vi "Read Measurement (Occupied Bandwidth).vi"(0 "VISA resource name":refnum<visa-resource-name>, 5 "Maximum Time (120000 ms)":i32=120000, 11 "error in (no error)":errorcluster) -> (4 "VISA resource name out":refnum<visa-resource-name>, 6 "Occupied Bandwidth(Hz)":dbl, 10 "Centroid Bandwidth(Hz)":dbl, 15 "error out":errorcluster)   [LabVIEW 2022 SP3, in "Agilent N934X Series.lvlib"]
doc: "Reads the measurement result from the spectrum analyzer (Occupied Bandwidth Measurement)."
uses:
  <instrlib>/Agilent N934X Series/Agilent N934X Series.lvlib
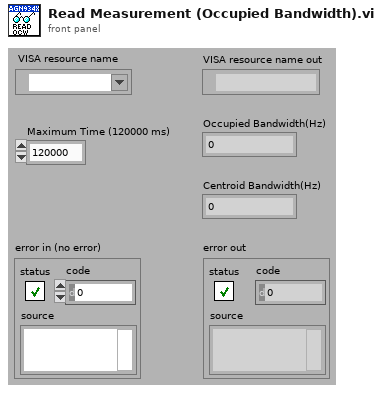
[diagram p1: front panel]
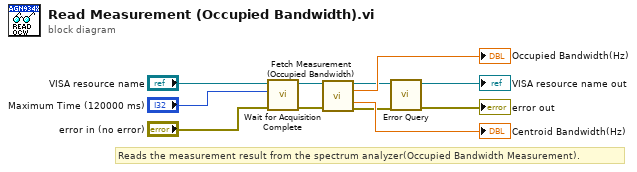
[diagram p0: block diagram]
diagram:
  # "Reads the measurement result from the spectrum analyzer(Occupied Bandwidth Measurement)."
  n1 = call <instrlib>:"Wait for Acquisition Complete.vi"("error in (no error)"="error in (no error)", "Maximum Time (10000 ms)"="Maximum Time (120000 ms)", "VISA resource name"="VISA resource name") -> ("error out"=w6:errorcluster, "VISA resource name out"=w8:refnum<visa-resource-name>)  [unwired: 7 in]
  n2 = call <instrlib>:"Fetch Measurement (Occupied Bandwidth).vi"("VISA resource name"=w8, "error in (no error)"=w6) -> ("VISA resource name out"=w4:refnum<visa-resource-name>, "Occupied Bandwidth(Hz)"=→"Occupied Bandwidth(Hz)":dbl, "Centroid Bandwidth(Hz)"=→"Centroid Bandwidth(Hz)":dbl, "error out"=w3:errorcluster)  [unwired: 10 in]
  n3 = call <instrlib>:"Error Query.vi"("error in (no error)"=w3, "VISA resource name"=w4) -> ("error out"=→"error out":errorcluster, "VISA resource name out"=→"VISA resource name out":refnum<visa-resource-name>)  [unwired: 6 in, 2 out]
